vi "Vibration Graph Screen.vi"() -> ()   [LabVIEW 2022 SP3]
uses:
  db641068-9fbb-4684-84d4-e9ad59cbcf60.vi
panel:
  out "Vertical":dbl[](graph)
  out "Horizontal 2":dbl[](graph)
  out "Axial 2":dbl[](graph)
  out "Vertical":dbl[](graph)
  out "Horizontal":dbl[](graph)
  out "Axial":dbl[](graph)
  out "error out":errorcluster
  in  "error in (no error)":errorcluster
  in  "Power Square":bool
  # "VIBRATION GRAPH SCREEN"
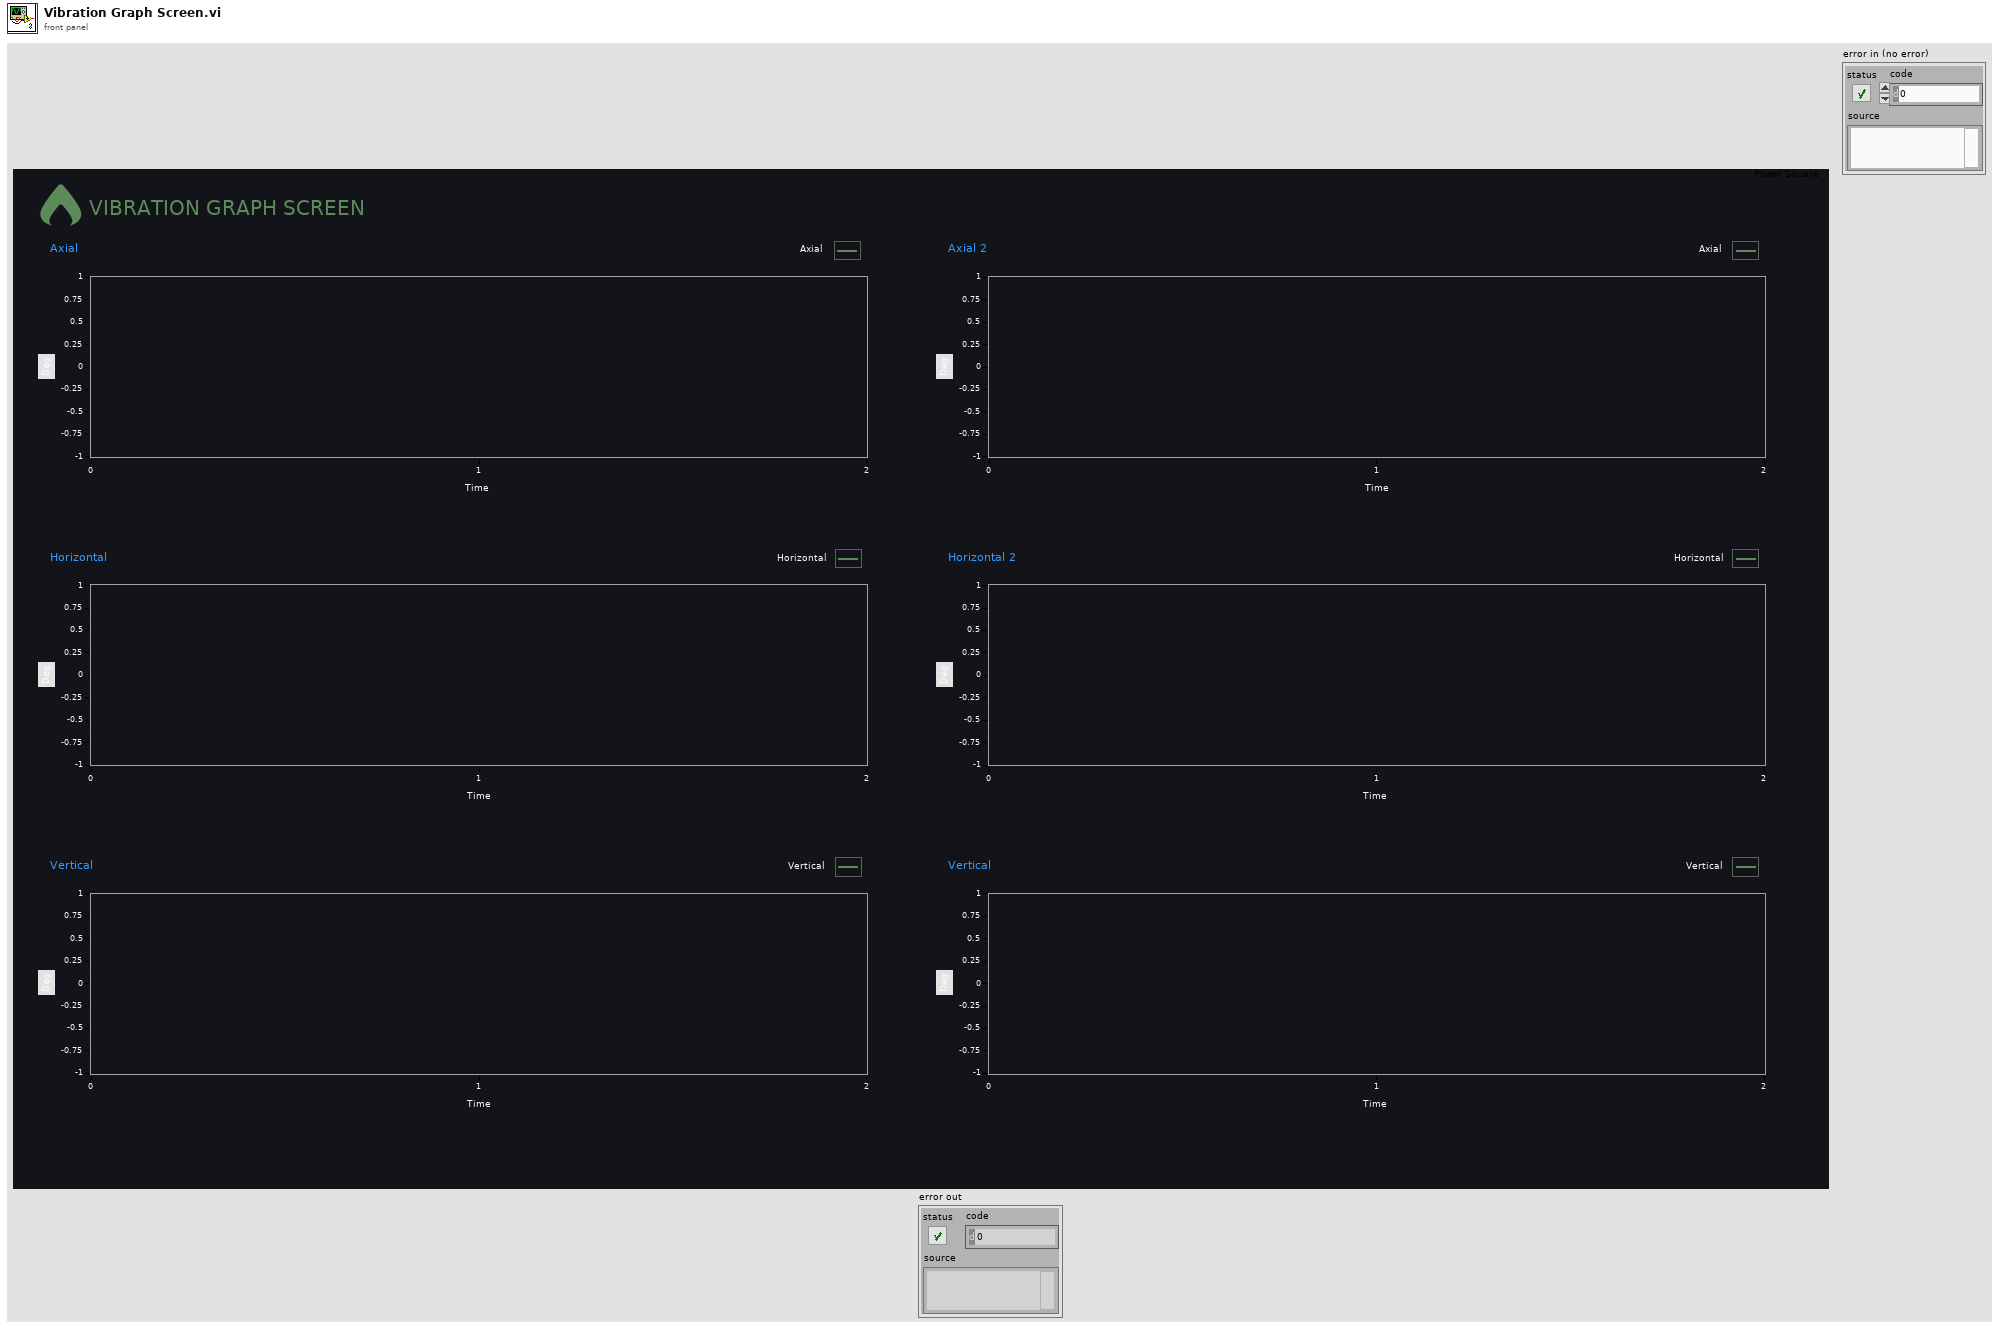
[diagram p1: front panel]
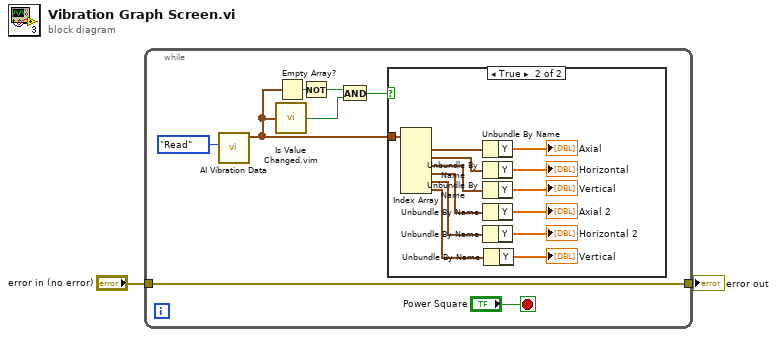
[diagram p0: block diagram]
diagram:
  n1 = while {
    tunnel: [w9] -> w1
    tunnel: "error in (no error)" -> [w9]
    stop <- "Power Square" stop-if-true
    n2 = call "AI Vibration Data.vi"("Enum"=enum16{"Read", "Write"}."Read") -> ("Vibration Data"=w3:waveform(dbl)[])  [unwired: 10 in]
    n3 = call "Is Value Changed.vim"("value"=w3) -> ("changed or first call?"=w6:bool)
    n4 = Empty Array?(array=w3) -> (empty?=w8:bool)
    n5 = Not(x=w8) -> (.not. x?=w7:bool)
    n6 = And(x=w7, y=w6) -> (x .and. y?=w5:bool)
    n7 = case shown="True" w5 {
      tunnel: w3 -> [_ w23]
      frame False {
      }
      frame True {
        n8 = Index Array(array=w23) -> (element #1=w22:waveform(dbl), element #2=w20:waveform(dbl), element #3=w19:waveform(dbl), element #4=w18:waveform(dbl), element #5=w17:waveform(dbl), element #6=w12:waveform(dbl))  [unwired: 6 in]
        n9 = Unbundle By Name(w22) -> ("Y"=→"Axial":dbl[])
        n10 = Unbundle By Name(w20) -> ("Y"=→"Horizontal":dbl[])
        n11 = Unbundle By Name(w19) -> ("Y"=→"Vertical":dbl[])
        n12 = Unbundle By Name(w18) -> ("Y"=→"Axial 2":dbl[])
        n13 = Unbundle By Name(w17) -> ("Y"=→"Horizontal 2":dbl[])
        n14 = Unbundle By Name(w12) -> ("Y"=→"Vertical":dbl[])
      }
    }
  }
  "error out" <- w1
